vi "lab session 8.2.vi"() -> ()   [LabVIEW 2020]
panel:
  in  "frequency":dbl
  in  "amplitude":dbl
  in  "stop":bool
  out "Waveform Chart":dynamicdata(graph)
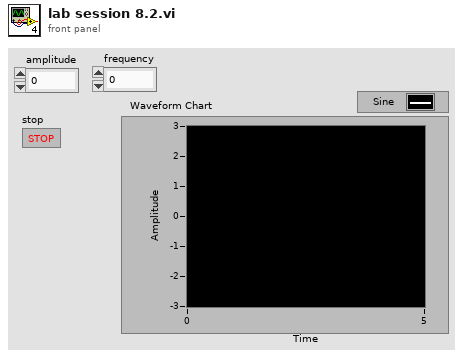
[diagram p1: front panel]
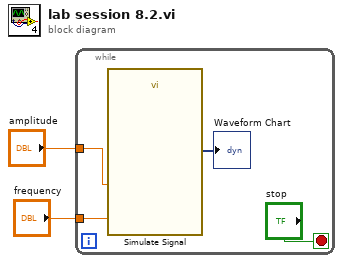
[diagram p0: block diagram]
diagram:
  n1 = while {
    tunnel: "amplitude" -> [w4]
    tunnel: "frequency" -> [w3]
    stop <- "stop" stop-if-true
    n2 = call "Simulate Signal"("Frequency"=w3, "Amplitude"=w4) -> ("Sine"=→"Waveform Chart":dynamicdata)  [unwired: 12 in, 1 out]
  }
